vi "Create External Network Setup Step.vi"(8 "error in (no error)":errorcluster, 10 "External Network Parameters":T1, 11 "QPA Measurement in":refnum<class "QPA Measurement.lvclass">=refnum) -> (0 "error out":errorcluster, 3 "QPA Measurement out":refnum<class "QPA Measurement.lvclass">)   [LabVIEW 2016, in "QPA Measurement.lvlib" / "QPA Measurement.lvclass"]
uses:
  QPA Measurement.lvclass
  Controls/External Network Parameters.ctl
  Controls/LoadPull State.ctl
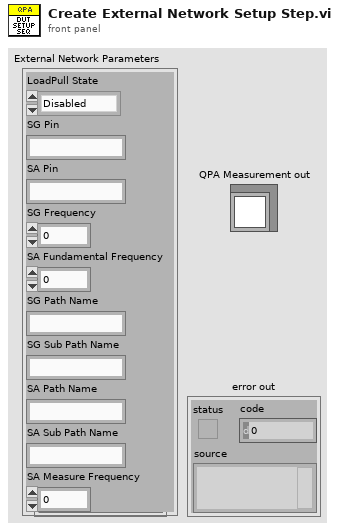
[diagram p1: front panel]
types:
  T1 = typedef "QPA Measurement.lvlib/QPA Measurement.lvclass/External Network Parameters.ctl" = cluster{"LoadPull State":T2, "SG Pin":string, "SA Pin":string, "SG Frequency":dbl, "SA Fundamental Frequency":dbl, "SG Path Name":string, "SG Sub Path Name":string, "SA Path Name":string, "SA Sub Path Name":string, "SA Measure Frequency":dbl}
  T2 = typedef "QPA Measurement.lvlib/QPA Measurement.lvclass/LoadPull State.ctl" = enum16{"Disabled", "Coupled Path", "Uncoupled Path", "Auto"}
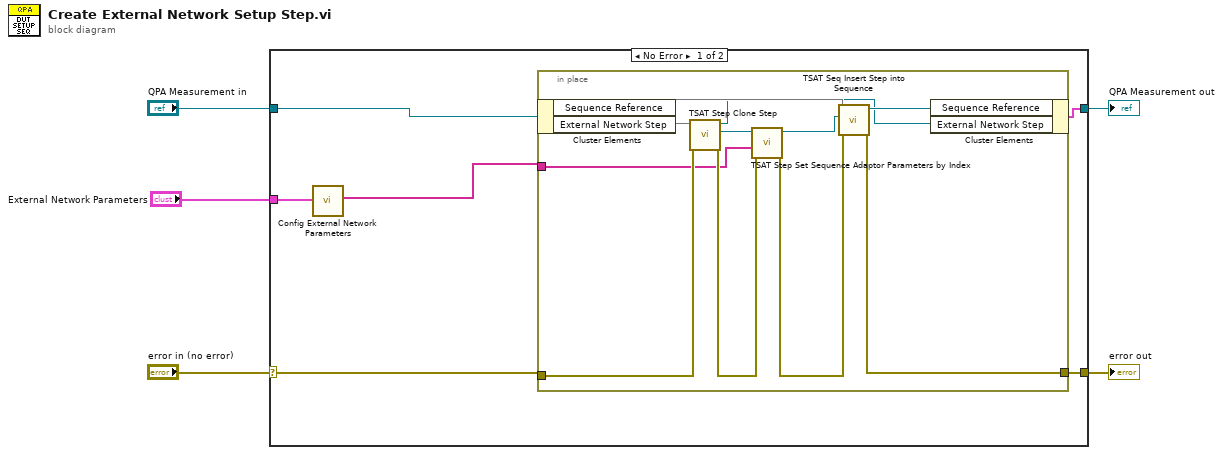
[diagram p0: block diagram]
diagram:
  n1 = case shown="No Error" "error in (no error)" {
    selector: "error in (no error)" -> [w11 w24]
    tunnel: [w8 w24] -> w4
    tunnel: [w10 w23] -> w2
    tunnel: "QPA Measurement in" -> [w9 w23]
    tunnel: "External Network Parameters" -> [w7 _]
    frame No Error {
      n2 = call "Config External Network Parameters.vi"("External Network Parameters"=w7) -> ("Parameters As Expressions"=w6:string[])  [unwired: 10 in]
      n3 = in-place {
        in-place-border: w11 -> [w18]
        in-place-border: w6 -> [w13]
        in-place-border: [w20] -> w8
        n4 = in-place-cluster #1(w9) -> ("Sequence Reference"=w22, "External Network Step"=w19)
        n5 = call "TSAT Step Clone Step.vi"("Error In"=w18, "Step In"=w19) -> ("Error Out"=w15:errorcluster, "Cloned Step"=w17:refnum<k7>, "Step Out"=w12:refnum<k7>)  [unwired: 7 in]
        n6 = call "TSAT Step Set Sequence Adaptor Parameters by Index.vi"("error in"=w15, "Parameter Array"=w13, "Step In"=w17) -> ("Error Out"=w14:errorcluster, "Step Out"=w16:refnum<k7>)  [unwired: 7 in]
        n7 = call "TSAT Seq Insert Step into Sequence.vi"("Error in"=w14, "Step to Add"=w16, "Sequence In"=w22) -> ("error out"=w20:errorcluster, "Sequence Out"=w21:refnum<k7>)  [unwired: 7 in]
        n8 = in-place-cluster #1("Sequence Reference"=w21, "External Network Step"=w12) -> (w10:cluster{})
      }
    }
    frame Error {
    }
  }
  "error out" <- w4
  "QPA Measurement out" <- w2
